vi "Get Result.vi"(8 "error in (no error)":errorcluster, 11 "Simple VISA Reader Driver in":refnum<class "Simple VISA Reader Driver.lvclass">) -> (0 "error out":errorcluster, 2 "Result":refnum<class "Acquired Result.lvclass">, 3 "Simple VISA Reader Driver out":refnum<class "Simple VISA Reader Driver.lvclass">)   [LabVIEW 2019, in "Simple VISA Reader Driver.lvclass"]
uses:
  Simple VISA Reader Driver.lvclass
  Results/Acquired Result/Acquired Result.lvclass
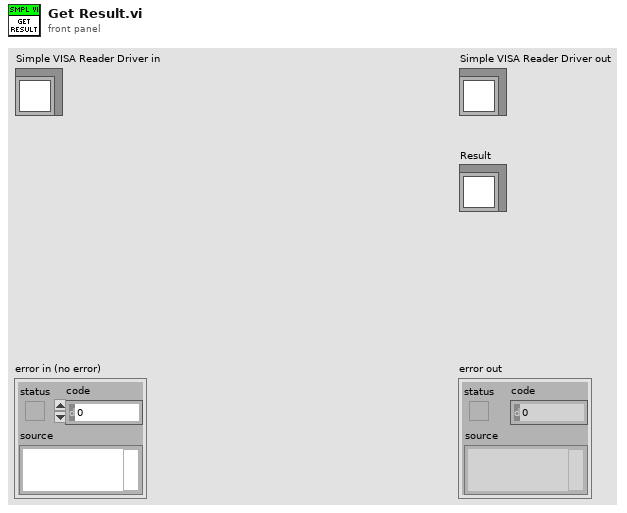
[diagram p1: front panel]
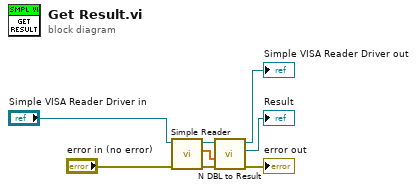
[diagram p0: block diagram]
diagram:
  n1 = call-dynamic "Simple Reader.vi"("error in (no error)"="error in (no error)", "Simple VISA Reader Driver in"="Simple VISA Reader Driver in") -> ("error out"=w2:errorcluster, "Signals"=w3:dbl[], "Simple VISA Reader Driver out"=w6:refnum<class "Simple VISA Reader Driver.lvclass">)  [unwired: 7 in]
  n2 = call-dynamic "N DBL to Result.vi"("error in (no error)"=w2, "Data"=w3, "Instrument Driver in"=w6) -> ("error out"=→"error out":errorcluster, "Result out"=→"Result":refnum<class "Acquired Result.lvclass">, "Instrument Driver out"=→"Simple VISA Reader Driver out":refnum<class "Simple VISA Reader Driver.lvclass">)  [unwired: 6 in]
